vi "Async Root.vi"(4 "UID":string, 10 "Root Actors":refnum<class "Root Actors.lvclass">) -> (0 "Error out":errorcluster, 2 "Root Attributes":refnum<class "Attributes.lvclass">)   [LabVIEW 2020, in "jettl.lvlib" / "Spawn.lvlib"]
uses:
  Spawn/Spawn.lvlib
  Attributes/Attributes.lvclass
  Root Actors/Root Actors.lvclass
  Attributes Metadata/Attributes Metadata.lvclass
  Actor/Actor.lvclass
  Transport/Transport.lvclass
  Msg/Msg.lvclass
  jettl.lvlib
  Base Attributes/Base Attributes.lvlib
  Msgs.ctl
  Attributes.ctl
  Lifetime.ctl
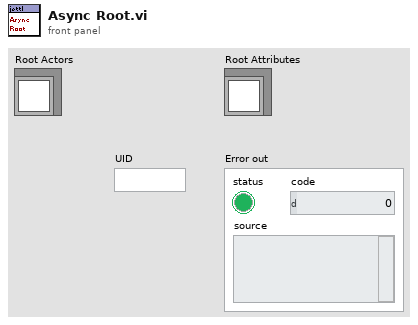
[diagram p1: front panel]
types:
  T1 = typedef "jettl.lvlib/Lifetime.ctl" = enum16{"Init", "Spawn", "Pre-Setup", "Setup", "Post-Setup", "Start", "Teardown", "Stopping With Children", "Stopping", "Stopped", "Terminate"}
  T2 = typedef "jettl.lvlib/Attributes.ctl" = cluster{"Attributes Metadata":refnum<class "Attributes Metadata.lvclass">, "Unified Msgs":T3, "Edge Actors":refnum<class "Actor.lvclass">[], "Core Actors":refnum<class "Actor.lvclass">[], "Parent Attributes":refnum<class "Attributes.lvclass">, "Root":bool, "UID":string, "Transport":refnum<class "Transport.lvclass">, "VI Ref":refnum<vi>, "Actors":refnum<class "Actor.lvclass">[]}
  T3 = typedef "jettl.lvlib/Msgs.ctl" = set{refnum<class "Msg.lvclass">}
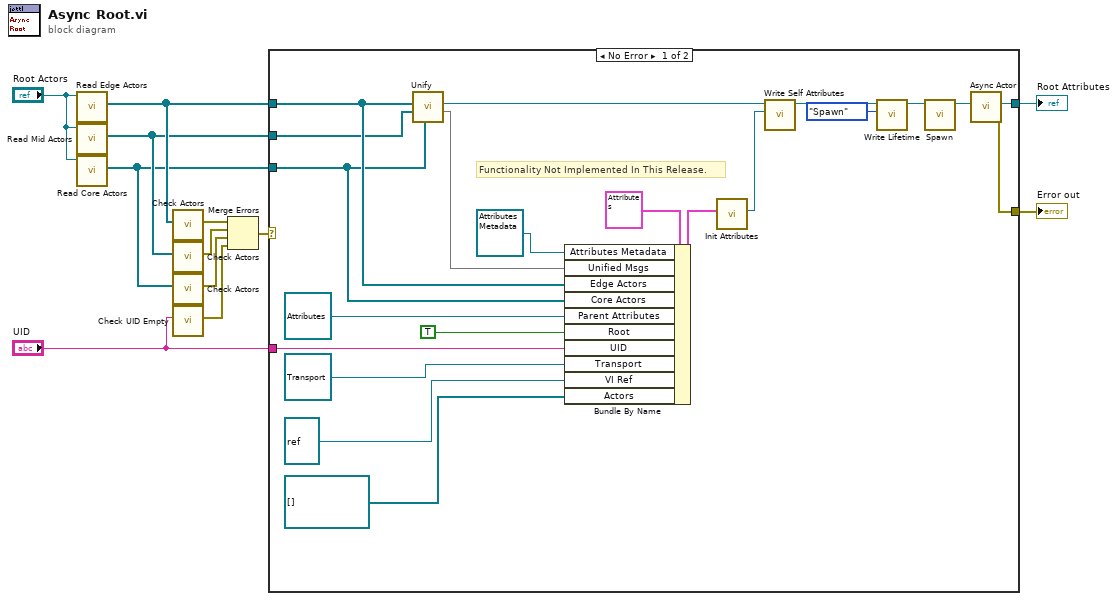
[diagram p0: block diagram]
diagram:
  n1 = call-dynamic "Read Edge Actors.vi"("Root Actors in"="Root Actors") -> ("Edge Actors"=w3:refnum<class "Actor.lvclass">[])  [unwired: 10 in]
  n2 = call-dynamic "Read Mid Actors.vi"("Root Actors in"="Root Actors") -> ("Mid Actors"=w2:refnum<class "Actor.lvclass">[])  [unwired: 10 in]
  n3 = call-dynamic "Read Core Actors.vi"("Root Actors in"="Root Actors") -> ("Core Actors"=w1:refnum<class "Actor.lvclass">[])  [unwired: 10 in]
  n4 = call "Check Actors.vi"("Actors"=w3) -> ("Error"=w5:errorcluster)  [unwired: 10 in]
  n5 = call "Check Actors.vi"("Actors"=w2) -> ("Error"=w9:errorcluster)  [unwired: 10 in]
  n6 = call "Check Actors.vi"("Actors"=w1) -> ("Error"=w6:errorcluster)  [unwired: 10 in]
  n7 = call "Check UID Empty.vi"("UID"="UID") -> ("Error"=w8:errorcluster)  [unwired: 10 in]
  n8 = Merge Errors(w5, w9, w6, w8) -> (w10:errorcluster)
  n9 = case shown="No Error" w10 {
    selector: w10 -> [_ w34]
    tunnel: w3 -> [w21 _]
    tunnel: [w33 w34] -> w12
    tunnel: [w32 _] -> w11
    tunnel: "UID" -> [w30 _]
    tunnel: w2 -> [w20 _]
    tunnel: w1 -> [w19 _]
    frame No Error {
      # "Functionality Not Implemented In This Release."
      n10 = call "Unify.vi"("Core Actors"=w19, "Mid Actors"=w20, "Edge Actors"=w21) -> ("Unified Msgs"=w17:T3, "Unified Actor"=w18:refnum<class "Actor.lvclass">)  [unwired: 7 in]
      n11 = Bundle By Name(cluster=T2 {"Attributes Metadata"=refnum, "Unified Msgs"={}, "Edge Actors"=[], "Core Actors"=[], "Parent Attributes"=refnum, "Root"=FALSE, "UID"="", "Transport"=refnum, "VI Ref"=refnum, "Actors"=[]} ("Attributes"), "Attributes Metadata"=refnum<class "Attributes Metadata.lvclass"> refnum, "Unified Msgs"=w17, "Edge Actors"=w21, "Core Actors"=w19, "Parent Attributes"=refnum<class "Attributes.lvclass"> refnum, "Root"=TRUE, "UID"=w30, "Transport"=refnum<class "Transport.lvclass"> refnum, "VI Ref"=refnum<vi> refnum ("Actor Ref"), "Actors"=refnum<class "Actor.lvclass">[] []) -> (w23:T2)
      n12 = call "Init Attributes.vi"("Attributes"=w23) -> ("Attributes"=w31:refnum<class "Attributes.lvclass">)  [unwired: 10 in]
      n13 = call-dynamic "Write Self Attributes.vi"("Self Attributes"=w31, "Actor in"=w18) -> ("Actor out"=w15:refnum<class "Actor.lvclass">)  [unwired: 9 in]
      n14 = call-dynamic "Write Lifetime.vi"("Lifetime"=Lifetime."Spawn", "Actor in"=w15) -> ("Actor out"=w14:refnum<class "Actor.lvclass">)  [unwired: 9 in]
      n15 = call-dynamic "Spawn.vi"("Actor in"=w14) -> ("Actor out"=w22:refnum<class "Actor.lvclass">)  [unwired: 10 in]
      n16 = call "Async Actor.vi"("Unified Actor"=w22) -> ("Error out"=w33:errorcluster, "Child Attributes"=w32:refnum<class "Attributes.lvclass">)  [unwired: 9 in]
    }
    frame Error {
    }
  }
  "Error out" <- w12
  "Root Attributes" <- w11
